vi "EditMoves.vi"() -> ()   [LabVIEW 2017]
uses:
  Auton.ctl
panel:
  in  "Cancel":bool
  in  "Team Number":i32=4810
  in  "Send":bool
  in  "Save":bool
  in  "Array":T1[](array[typedef])
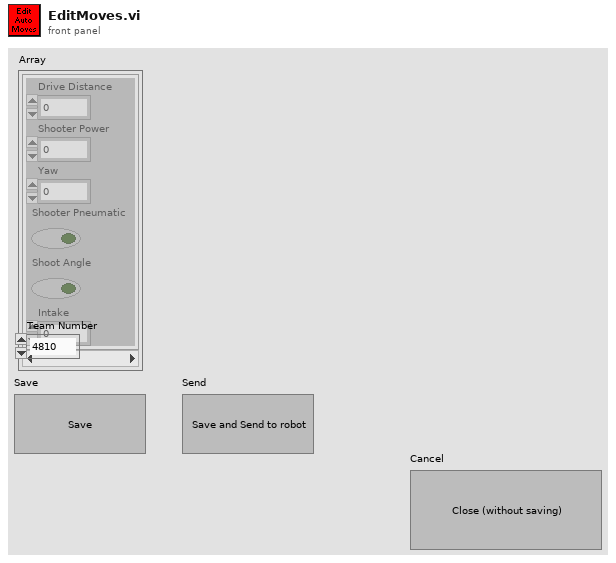
[diagram p1: front panel]
types:
  T1 = typedef "Auton.ctl" = cluster{"Drive Distance":dbl, "Shooter Power":dbl, "Yaw":dbl, "Shooter Pneumatic":bool, "Shoot Angle":bool, "Intake":dbl}
  T2 = enum16{"Init", "Save locally", "Update Cache", "Send to Bot", "Waiting"}
  T3 = enum16{"open", "replace", "create", "open or create", "replace or create", "replace or create with confirmation"}
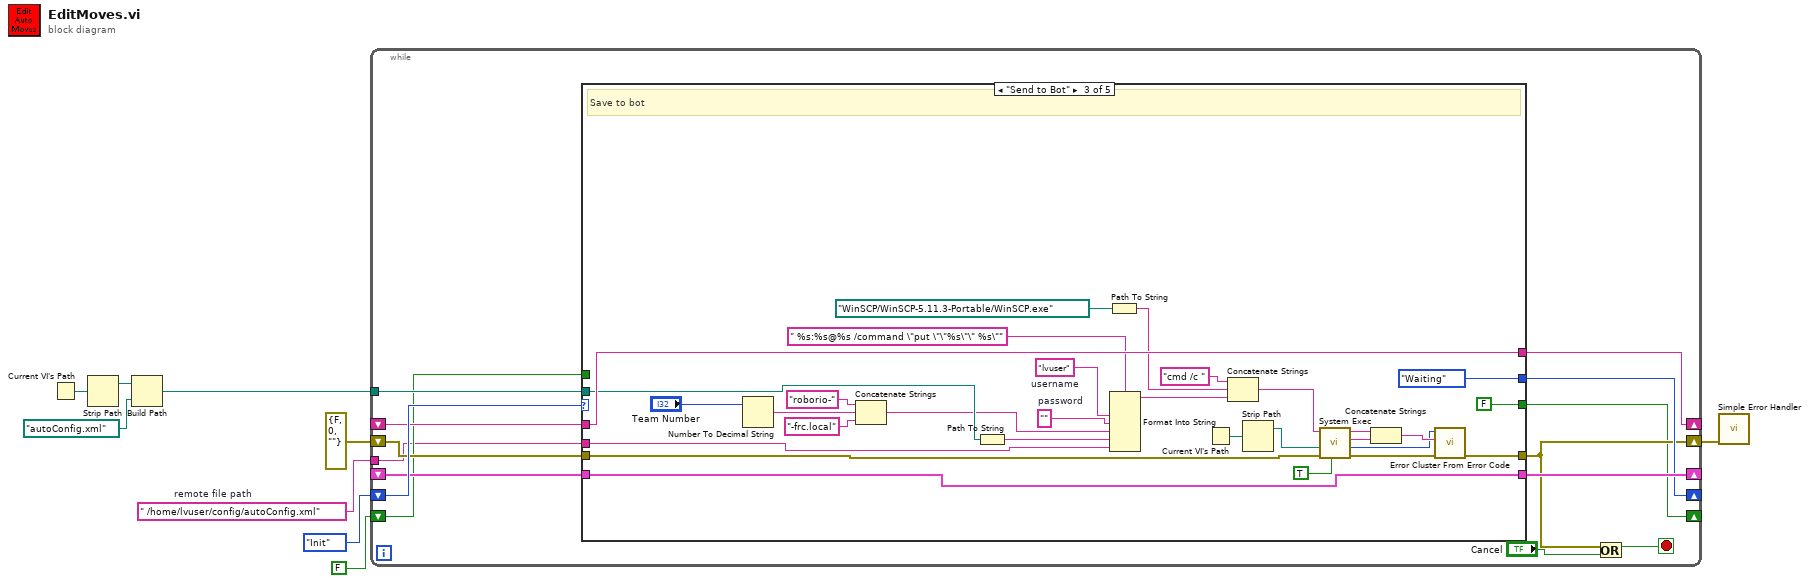
[diagram p0: block diagram]
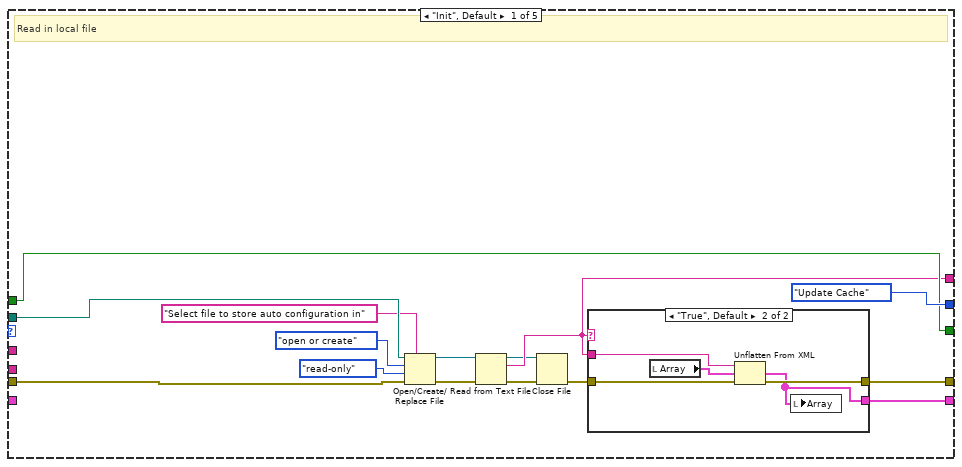
[diagram p2: hidden frame]
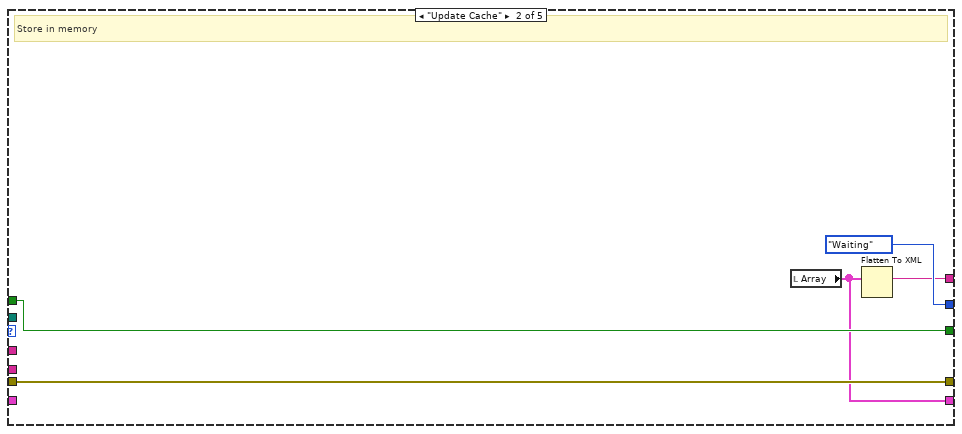
[diagram p4: hidden frame]
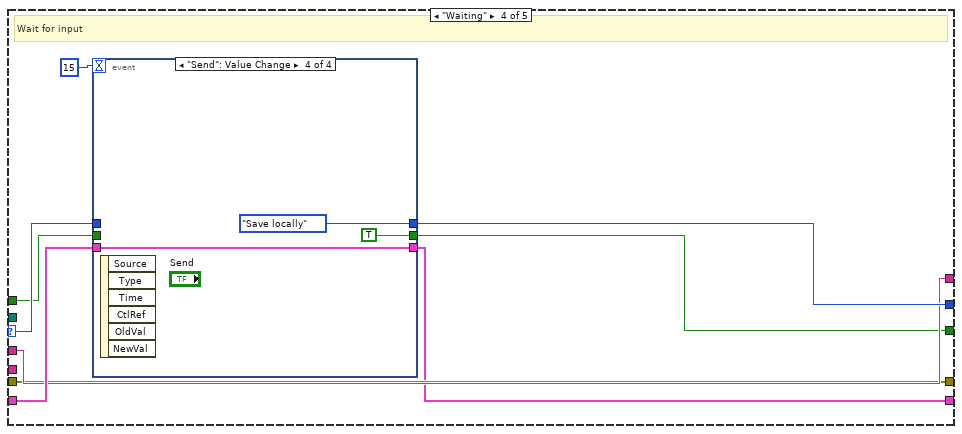
[diagram p5: hidden frame]
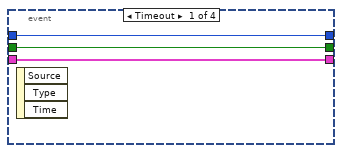
[diagram p6: hidden frame]
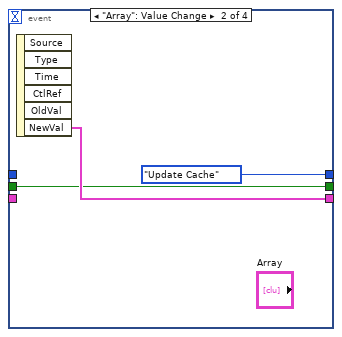
[diagram p7: hidden frame]
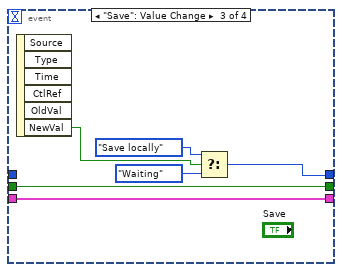
[diagram p8: hidden frame]
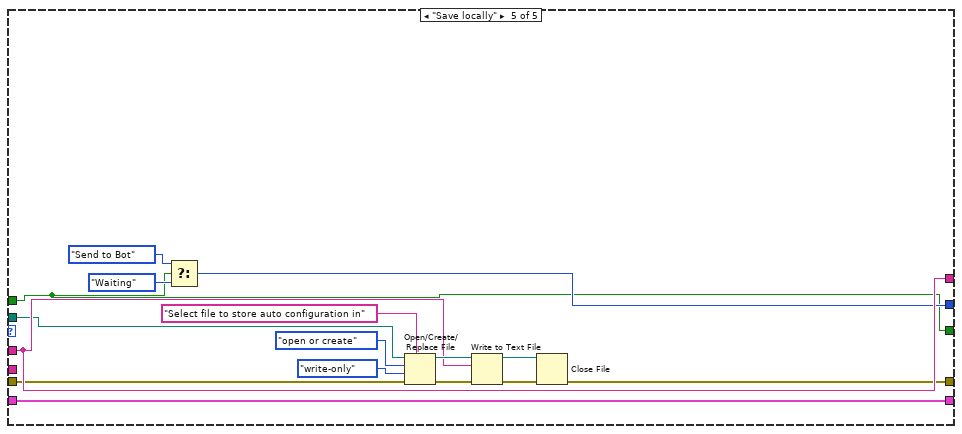
[diagram p9: hidden frame]
diagram:
  w1 = " /home/lvuser/config/autoConfig.xml"  # remote file path
  n1 = Current VI's Path() -> (path=w6:path)
  n2 = Strip Path(path=w6) -> (stripped path=w5:path)  [unwired: 1 out]
  n3 = Build Path(base path=w5, name or relative path=path "autoConfig.xml" ("file path (use dialog)")) -> (appended path=w3:path)
  n4 = while {
    shift-right: [w21] -> _
    shift-left: T2."Init" -> [w23]
    shift-right: [w22] -> _
    shift-left: _ -> [w20]
    shift-right: [w19] -> _
    shift-left: _ -> [w15]
    shift-right: [w18] -> w7
    shift-left: errorcluster {"status"=FALSE, "code"=0, "source"=""} ("error out") -> [w16]
    tunnel: w3 -> [w17]
    shift-right: [w13] -> _
    shift-left: FALSE -> [w14]
    tunnel: w1 -> [w12]
    stop <- w11 stop-if-true
    n5 = case shown="\"Send to Bot\"" w23 {
      selector: w23 -> [_ _ _ w86 _]
      tunnel: [w24 w45 w79 w80 w119] -> w22
      tunnel: [T2."Update Cache" T2."Waiting" T2."Waiting" w88 w108] -> w21
      tunnel: w20 -> [_ _ w79 w87 w119]
      tunnel: [w32 w46 w78 w84 w111] -> w19
      tunnel: [w35 w47 w70 w83 w106] -> w18
      tunnel: w17 -> [w34 _ w74 _ w104]
      tunnel: w16 -> [w33 w47 w73 w83 w105]
      tunnel: w15 -> [_ _ w78 w84 w111]
      tunnel: w14 -> [w37 w48 _ w81 w107]
      tunnel: [w37 w48 FALSE w82 w107] -> w13
      tunnel: w12 -> [_ _ w59 _ _]
      frame "Init", Default {
        # "Read in local file"
        n6 = Open/Create/Replace File(file path (use dialog)=w34, error in=w33, prompt="Select file to store auto configuration in", operation (0:open)=T3."open or create", access (0:read/write)=enum16{"read/write", "read-only", "write-only"}."read-only") -> (refnum out=w28:refnum<file>, error out=w27:errorcluster)  [unwired: 1 in, 1 out]
        n7 = Read from Text File(file (use dialog)=w28, error in=w27) -> (refnum out=w25:refnum<file>, text=w32:string, error out=w26:errorcluster)  [unwired: 2 in, 1 out]
        n8 = Close File(refnum=w25, error in=w26) -> (error out=w36:errorcluster)  [unwired: 1 out]
        n9 = case shown="\"True\", Default" w32 {
          tunnel: w32 -> [_ w44]
          tunnel: w36 -> [w39 w42]
          tunnel: [w39 w41] -> w35
          tunnel: [_ w40] -> w24
          frame "" {
          }
          frame "True", Default {
            n10 = local read "Array"() -> (w43:T1[])
            n11 = Unflatten From XML(xml string=w44, type=w43, error in (no error)=w42) -> (value=w40:T1[], error out=w41:errorcluster)
            n12 = local write "Array"(w40) -> ()
          }
        }
      }
      frame "Update Cache" {
        # "Store in memory"
        n13 = local read "Array"() -> (w45:T1[])
        n14 = Flatten To XML(anything=w45) -> (xml string=w46:string)
      }
      frame "Send to Bot" {
        w63 = ""  # password
        w64 = "lvuser"  # username
        # "Save to bot"
        n15 = Number To Decimal String(number="Team Number") -> (decimal integer string=w50:string)  [unwired: 1 in]
        n16 = Concatenate Strings("roborio-" ("string"), w50, "-frc.local" ("string")) -> (w62:string)
        n17 = Path To String(path=w74) -> (string=w61:string)
        n18 = Path To String(path=path "WinSCP/WinSCP-5.11.3-Portable/WinSCP.exe") -> (string=w54:string)
        n19 = Format Into String(format string=" %s:%s@%s /command \"put \"\"%s\"\" %s\"", w64, w63, w62, w61, w59) -> (resulting string=w60:string)  [unwired: 2 in, 1 out]
        n20 = Current VI's Path() -> (path=w75:path)
        n21 = Concatenate Strings("cmd /c " ("string"), w54, w60) -> (w56:string)
        n22 = Strip Path(path=w75) -> (stripped path=w65:path)  [unwired: 1 out]
        n23 = call <vilib>:"System Exec.vi"("run minimized? (F)"=TRUE, "error in (no error)"=w73, "working directory"=w65, "command line"=w56) -> ("error out"=w71:errorcluster, "return code"=w66:i32, "standard error"=w67:string, "standard output"=w68:string)  [unwired: 4 in]
        n24 = Concatenate Strings(w68, w67) -> (w69:string)
        n25 = call <vilib>:"Error Cluster From Error Code.vi"("error in (no error)"=w71, "error message (\"\")"=w69, "error code (0)"=w66) -> ("error out"=w70:errorcluster)  [unwired: 6 in]
      }
      frame "Waiting" {
        # "Wait for input"
        n26 = event shown="[3] \"Send\": Value Change" {
          selector: _ -> [_ _ _ _]
          dyn-events: _ -> [_ _ _ _]
          timeout: 15 -> [_ _ _ _]
          tunnel: [w89 w94 w95 w101] -> w80
          tunnel: [w91 T2."Update Cache" w99 T2."Save locally"] -> w88
          tunnel: w87 -> [w89 _ w95 w101]
          tunnel: w86 -> [w91 _ _ _]
          tunnel: [w90 w92 w96 TRUE] -> w82
          tunnel: w81 -> [w90 w92 w96 _]
          event Timeout {
            n27 = event-data() -> ()  [unwired: 1 in, 3 out]
          }
          event "Array": Value Change {
            n28 = event-data() -> ("NewVal"=w94:T1[])  [unwired: 1 in, 5 out]
          }
          event "Save": Value Change {
            n29 = event-data() -> ("NewVal"=w100:bool)  [unwired: 1 in, 5 out]
            n30 = Select(t=T2."Save locally", s=w100, f=T2."Waiting") -> (s? t:f=w99:T2)
          }
          event "Send": Value Change {
            n31 = event-data() -> ()  [unwired: 1 in, 6 out]
          }
        }
      }
      frame "Save locally" {
        n32 = Select(t=T2."Send to Bot", s=w107, f=T2."Waiting") -> (s? t:f=w108:T2)
        n33 = Open/Create/Replace File(file path (use dialog)=w104, error in=w105, prompt="Select file to store auto configuration in", operation (0:open)=T3."open or create", access (0:read/write)=enum16{"read/write", "read-only", "write-only"}."write-only") -> (refnum out=w115:refnum<file>, error out=w114:errorcluster)  [unwired: 1 in, 1 out]
        n34 = Write to Text File(file (use dialog)=w115, text=w111, error in=w114) -> (refnum out=w112:refnum<file>, error out=w113:errorcluster)  [unwired: 1 in, 1 out]
        n35 = Close File(refnum=w112, error in=w113) -> (error out=w106:errorcluster)  [unwired: 1 out]
      }
    }
    n36 = Or(x=w18, y="Cancel") -> (x .or. y?=w11:bool)
  }
  n37 = call <vilib>:"Simple Error Handler.vi"("error in (no error)"=w7) -> ()  [unwired: 4 in, 5 out]
